vi "Configurator.vi"() -> ()   [LabVIEW 2017]
uses:
  Controls/Configurator Range Enum Type Def.ctl
  Controls/Configurator Rate Enum Type Def.ctl
  Controls/xlRange.ctl
panel:
  in  "Accelerometer Range":T1=enum."±8g"
  in  "First Erase?":bool
  in  "VISA":refnum<visa-resource-name>
  out "Error Out":errorcluster
  in  "Error In":errorcluster
  in  "ID":u8
  in  "Rate":T2=enum."52"
  in  "Angular Velocity Range":T3=enum."250 dps"
  # "Read and save measurement data before running this program!"
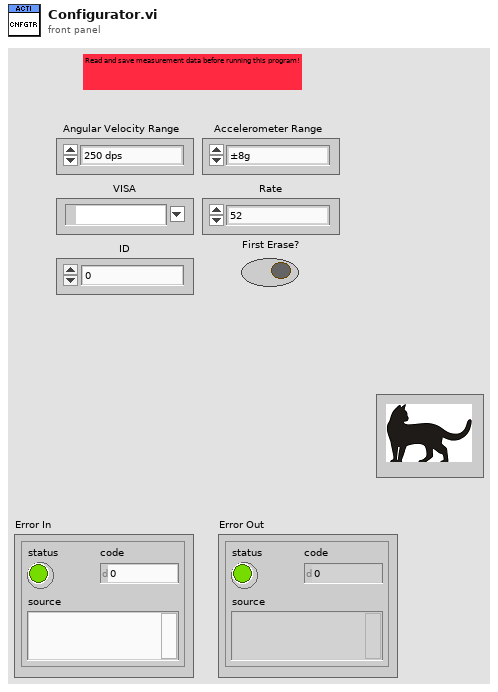
[diagram p1: front panel]
types:
  T1 = typedef "xlRange.ctl" = enum16{"±16g", "±8g", "±4g", "±2g"}
  T2 = typedef "Configurator Rate Enum Type Def.ctl" = enum16{"12,5", "208", "104", "52", "26", "Idle"}
  T3 = typedef "Configurator Range Enum Type Def.ctl" = enum16{"125 dps", "250 dps", "500 dps", "1000 dps", "2000 dps", ""}
  T4 = cluster{"Angular Velocity Range":T3, "Accelerometer Range":T1, "ID":u8, "VISA":refnum<visa-resource-name>, "First Erase?":bool, "xlRange":u8, "gyroRange":u8, "ODR":u8, "Time Bytes":string, "Rate":T2}
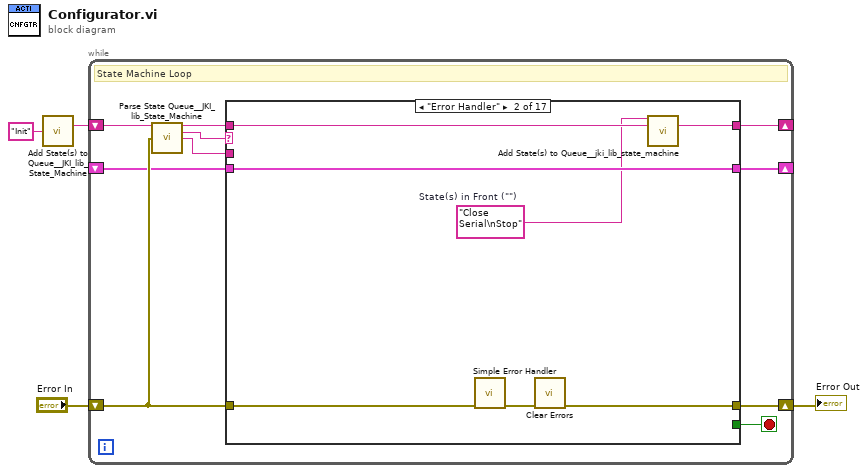
[diagram p0: block diagram]
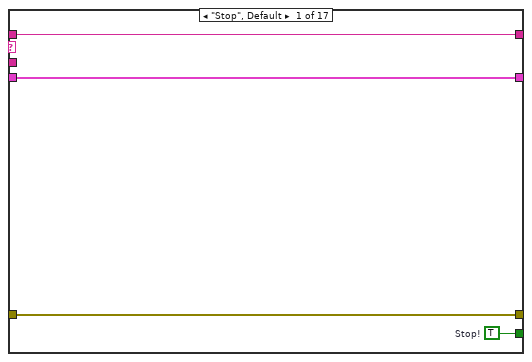
[diagram p2: hidden frame]
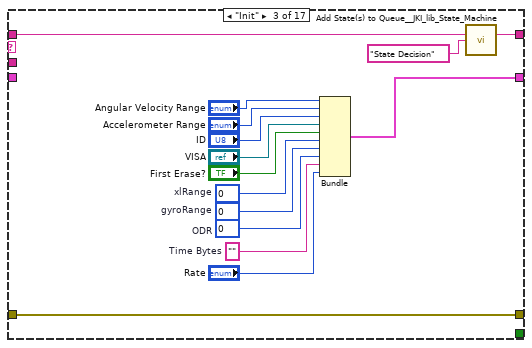
[diagram p3: hidden frame]
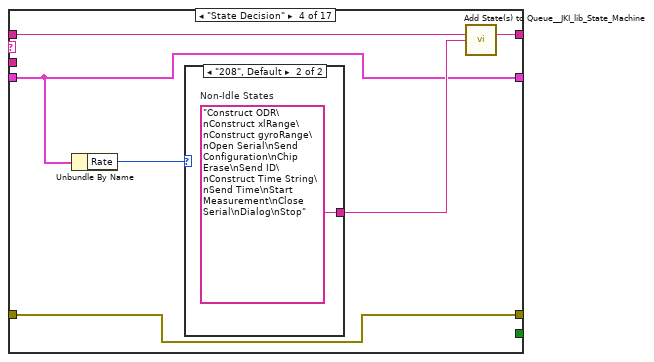
[diagram p4: hidden frame]
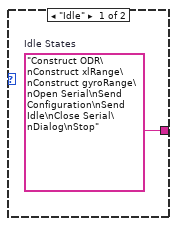
[diagram p5: hidden frame]
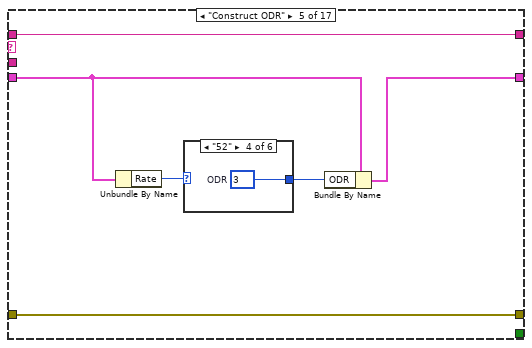
[diagram p6: hidden frame]
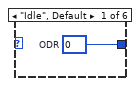
[diagram p7: hidden frame]
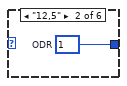
[diagram p8: hidden frame]
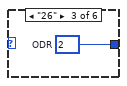
[diagram p9: hidden frame]
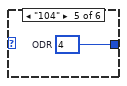
[diagram p10: hidden frame]
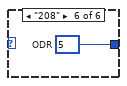
[diagram p11: hidden frame]
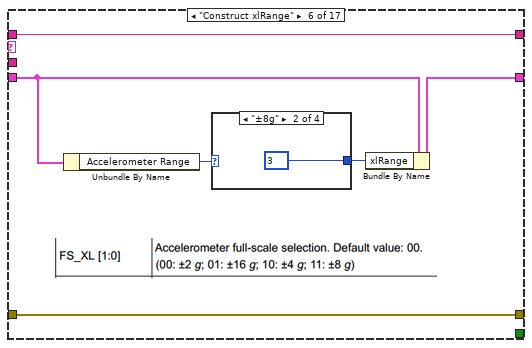
[diagram p12: hidden frame]
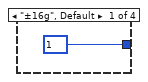
[diagram p13: hidden frame]
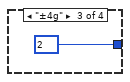
[diagram p14: hidden frame]
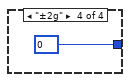
[diagram p15: hidden frame]
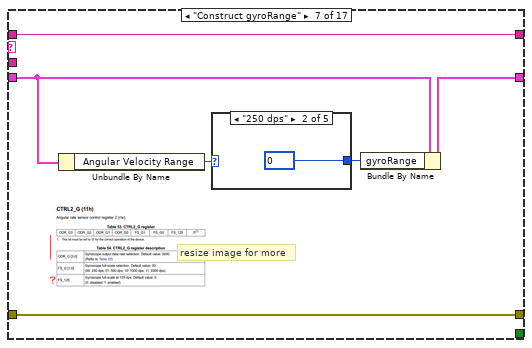
[diagram p16: hidden frame]
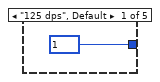
[diagram p17: hidden frame]
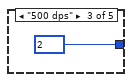
[diagram p18: hidden frame]
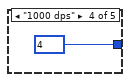
[diagram p19: hidden frame]
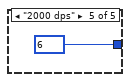
[diagram p20: hidden frame]
diagram:
  n1 = call <vilib>:"Add State(s) to Queue__JKI_lib_State_Machine.vi"("State(s) at Back (\"\")"="Init" ("State(s) at Back (\"\")")) -> ("States Out"=w2:string)  [unwired: 14 in]
  n2 = while {
    shift-right: [w13] -> w3
    shift-left: "Error In" -> [w14]
    shift-right: [w11] -> _
    shift-left: _ -> [w10]
    shift-right: [w6] -> _
    shift-left: w2 -> [w9]
    stop <- w12 stop-if-true
    # "State Machine Loop"
    n3 = call <vilib>:"Parse State Queue__JKI_lib_State_Machine.vi"("State Queue"=w9, "Error In (no error)"=w14) -> ("Remaining States"=w5:string, "Current State"=w8:string, "Arguments"=w7:string)  [unwired: 11 in]
    n4 = case shown="\"Error Handler\"" w8 {
      tunnel: w14 -> [w16 w25 w40 w42 w54 w66 w76 w87 w93 w114 w130 w140 w151 w157 w162 w175 w182]
      tunnel: [w16 w19 w40 w42 w54 w66 w76 w86 w100 w112 w122 w139 w150 w156 w161 w175 w182] -> w13
      tunnel: [w18 _ _ _ _ _ _ _ _ _ _ _ _ _ _ _ _] -> w12
      tunnel: [w17 w24 w31 w41 w50 w64 w74 w85 w101 w104 w129 w136 w149 w155 w160 w177 w180] -> w11
      tunnel: w10 -> [w17 w24 _ w41 w51 w65 w75 w85 w101 w104 w129 w143 w149 w155 w160 w177 w180]
      tunnel: w7 -> [_ _ _ _ _ _ _ _ _ _ _ _ _ _ _ _ _]
      tunnel: [w15 w23 w29 w46 w53 w63 w73 w83 w97 w102 w120 w132 w144 w152 w158 w174 w178] -> w6
      tunnel: w5 -> [w15 w22 w28 w45 w53 w63 w73 w83 w97 w102 w120 w132 w144 w152 w158 w174 w178]
      frame "Stop", Default {
        w18 = TRUE  # Stop!
      }
      frame "Error Handler" {
        w21 = "Close Serial\nStop"  # State(s) in Front ("")
        n5 = call <vilib>:"Simple Error Handler.vi"("error in (no error)"=w25) -> ("error out"=w20:errorcluster)  [unwired: 4 in, 4 out]
        n6 = call <vilib>:"Clear Errors.vi"("error in (no error)"=w20) -> ("error out"=w19:errorcluster)  [unwired: 5 in, 1 out]
        n7 = call <vilib>:"Add State(s) to Queue__jki_lib_state_machine.vi"("State(s) in Front (\"\")"=w21, "State(s) in (\"\")"=w22) -> ("States Out"=w23:string)  [unwired: 13 in]
      }
      frame "Init" {
        w30 = u8 0  # gyroRange
        w32 = ""  # Time Bytes
        w33 = u8 0  # ODR
        w34 = u8 0  # xlRange
        n8 = Bundle("Angular Velocity Range"="Angular Velocity Range", "Accelerometer Range"="Accelerometer Range", "ID"="ID", "VISA"="VISA", "First Erase?"="First Erase?", "xlRange"=w34, "gyroRange"=w30, "ODR"=w33, "Time Bytes"=w32, "Rate"="Rate") -> (w31:T4)  [unwired: 1 in]
        n9 = call <vilib>:"Add State(s) to Queue__JKI_lib_State_Machine.vi"("State(s) in (\"\")"=w28, "State(s) at Back (\"\")"="State Decision" ("State(s) at Back (\"\")")) -> ("States Out"=w29:string)  [unwired: 13 in]
      }
      frame "State Decision" {
        n10 = Unbundle By Name(w41) -> ("Rate"=w44:T2)
        n11 = case shown="\"208\", Default" w44 {
          tunnel: [w47 w48] -> w43
          frame "Idle" {
            w47 = "Construct ODR\nConstruct xlRange\nConstruct gyroRange\nOpen Serial\nSend Configuration\nSend Idle\nClose Serial\nDialog\nStop"  # Idle States
          }
          frame "208", Default {
            w48 = "Construct ODR\nConstruct xlRange\nConstruct gyroRange\nOpen Serial\nSend Configuration\nChip Erase\nSend ID\nConstruct Time String\nSend Time\nStart Measurement\nClose Serial\nDialog\nStop"  # Non-Idle States
          }
        }
        n12 = call <vilib>:"Add State(s) to Queue__JKI_lib_State_Machine.vi"("State(s) in (\"\")"=w45, "State(s) at Back (\"\")"=w43) -> ("States Out"=w46:string)  [unwired: 13 in]
      }
      frame "Construct ODR" {
        n13 = Unbundle By Name(w51) -> ("Rate"=w52:T2)
        n14 = case shown="\"52\"" w52 {
          tunnel: [w55 w56 w57 w58 w59 w60] -> w49
          frame "Idle", Default {
            w55 = u8 0  # ODR
          }
          frame "12,5" {
            w56 = u8 1  # ODR
          }
          frame "26" {
            w57 = u8 2  # ODR
          }
          frame "52" {
            w58 = u8 3  # ODR
          }
          frame "104" {
            w59 = u8 4  # ODR
          }
          frame "208" {
            w60 = u8 5  # ODR
          }
        }
        n15 = Bundle By Name(cluster=w51, "ODR"=w49) -> (w50:T4)
      }
      frame "Construct xlRange" {
        n16 = Unbundle By Name(w65) -> ("Accelerometer Range"=w62:T1)
        n17 = case shown="\"±8g\"" w62 {
          tunnel: [u8 1 u8 3 u8 2 u8 0] -> w61
          frame "±16g", Default {
          }
          frame "±8g" {
          }
          frame "±4g" {
          }
          frame "±2g" {
          }
        }
        n18 = Bundle By Name(cluster=w65, "xlRange"=w61) -> (w64:T4)
      }
      frame "Construct gyroRange" {
        # "resize image for more"
        n19 = Unbundle By Name(w75) -> ("Angular Velocity Range"=w72:T3)
        n20 = case shown="\"250 dps\"" w72 {
          tunnel: [u8 1 u8 0 u8 2 u8 4 u8 6] -> w71
          frame "125 dps", Default {
          }
          frame "250 dps" {
          }
          frame "500 dps" {
          }
          frame "1000 dps" {
          }
          frame "2000 dps" {
          }
        }
        n21 = Bundle By Name(cluster=w75, "gyroRange"=w71) -> (w74:T4)
      }
      frame "Open Serial" {
        w82 = u32 6000000  # Baud rate
        n22 = Unbundle By Name(w85) -> ("VISA"=w84:refnum<visa-resource-name>)
        n23 = call "Init_VSP.vi"("error in"=w87, "Baud rate"=w82, "VISA resource name"=w84) -> ("error out"=w86:errorcluster)  [unwired: 7 in, 1 out]
      }
      frame "Send Configuration" {
        w90 = FALSE  # Prepend Size?
        w88 = "*C"  # Configure Command
        n24 = Unbundle By Name(w101) -> ("VISA"=w99:refnum<visa-resource-name>, "ODR"=w94:u8, "xlRange"=w96:u8, "gyroRange"=w95:u8)
        n25 = Build Array(w94, w96, w95) -> (w91:u8[])
        n26 = Flatten To String(anything=w91, prepend array or string size? (T)=w90, error in (no error)=w93) -> (data string=w89:string, error out=w92:errorcluster)  [unwired: 1 in, 1 out]
        n27 = Concatenate Strings(w88, w89) -> (w98:string)
        n28 = call "Write Serial One by One With Echo.vi"("String"=w98, "Error In"=w92, "VISA In"=w99) -> ("Error Out"=w100:errorcluster)  [unwired: 7 in, 1 out]
      }
      frame "Chip Erase" {
        w108 = "*1*Y"  # First Erase
        w107 = "*Y"  # Chip Erase Command
        n29 = Unbundle By Name(w104) -> ("First Erase?"=w103:bool)
        n30 = Unbundle By Name(w104) -> ("VISA"=w106:refnum<visa-resource-name>)
        n31 = Select(t=w108, s=w103, f=w107) -> (s? t:f=w105:string)
        n32 = call "Write Serial One by One With Echo.vi"("String"=w105, "Error In"=w114, "VISA In"=w106) -> ("Error Out"=w113:errorcluster, "VISA Out"=w110:refnum<visa-resource-name>)  [unwired: 7 in]
        n33 = for {
          N: 4 -> [_]
          shift-right: [w118] -> w112
          shift-left: w113 -> [w119]
          tunnel: u32 1 ("Requested byte cout") -> [w117]
          tunnel: w110 -> [w116]
          tunnel: [w115] -> _ mode=indexing
          n34 = call "Read_VSP.vi"("error in"=w119, "Requested byte count"=w117, "VISA resource name"=w116) -> ("error out"=w118:errorcluster, "String"=w115:string)  [unwired: 1 in, 2 out]
        }
      }
      frame "Send ID" {
        w126 = FALSE  # Prepend Size?
        w131 = "*D"  # Send ID Command
        n35 = Unbundle By Name(w129) -> ("ID"=w121:u8, "VISA"=w128:refnum<visa-resource-name>)
        n36 = call "Write Serial One by One With Echo.vi"("String"=w131, "Error In"=w130, "VISA In"=w128) -> ("Error Out"=w127:errorcluster, "VISA Out"=w124:refnum<visa-resource-name>)  [unwired: 7 in]
        n37 = Flatten To String(anything=w121, prepend array or string size? (T)=w126, error in (no error)=w127) -> (data string=w123:string, error out=w125:errorcluster)  [unwired: 1 in, 1 out]
        n38 = call "Write_VSP.vi"("error in"=w125, "String"=w123, "VISA resource name"=w124) -> ("error out"=w122:errorcluster)  [unwired: 2 in, 2 out]
      }
      frame "Construct Time String" {
        w133 = 4 ("offset (0)")
        w137 = FALSE  # Prepend Size?
        n39 = Get Date/Time In Seconds() -> (seconds since 1Jan1904=w142:timestamp)
        n40 = To Double Precision Float(number=w142) -> (double precision float=w141:dbl)
        n41 = To Unsigned Quad Integer(1:w141) -> (0:w138:u64)
        n42 = Flatten To String(anything=w138, prepend array or string size? (T)=w137, error in (no error)=w140) -> (data string=w134:string, error out=w139:errorcluster)  [unwired: 1 in, 1 out]
        n43 = String Subset(string=w134, offset (0)=w133, length (rest)=w133) -> (substring=w135:string)
        n44 = Bundle By Name(cluster=w143, "Time Bytes"=w135) -> (w136:T4)
      }
      frame "Send Time" {
        w148 = "*T"  # Set Time Command
        n45 = Unbundle By Name(w149) -> ("Time Bytes"=w147:string, "VISA"=w146:refnum<visa-resource-name>)
        n46 = Concatenate Strings(w148, w147) -> (w145:string)
        n47 = call "Write Serial One by One With Echo.vi"("String"=w145, "Error In"=w151, "VISA In"=w146) -> ("Error Out"=w150:errorcluster)  [unwired: 7 in, 1 out]
      }
      frame "Start Measurement" {
        w153 = "*S"  # Start Command
        n48 = Unbundle By Name(w155) -> ("VISA"=w154:refnum<visa-resource-name>)
        n49 = call "Write Serial One by One With Echo.vi"("String"=w153, "Error In"=w157, "VISA In"=w154) -> ("Error Out"=w156:errorcluster)  [unwired: 7 in, 1 out]
      }
      frame "Send Idle" {
        w164 = u8 27  # Esc Character
        w165 = u32 1  # Requested byte cout
        n50 = Unbundle By Name(w160) -> ("VISA"=w159:refnum<visa-resource-name>)
        n51 = call "Write_VSP.vi"("error in"=w162, "String"="*", "VISA resource name"=w159) -> ("error out"=w171:errorcluster, "duplicate VISA resource name"=w170:refnum<visa-resource-name>)  [unwired: 2 in, 1 out]
        n52 = Flatten To String(anything=w164) -> (data string=w163:string)  [unwired: 3 in, 2 out]
        n53 = call "Read_VSP.vi"("error in"=w171, "Requested byte count"=w165, "VISA resource name"=w170) -> ("error out"=w167:errorcluster, "duplicate VISA resource name"=w166:refnum<visa-resource-name>)  [unwired: 1 in, 2 out]
        n54 = call "Write_VSP.vi"("error in"=w167, "String"=w163, "VISA resource name"=w166) -> ("error out"=w168:errorcluster, "duplicate VISA resource name"=w169:refnum<visa-resource-name>)  [unwired: 2 in, 1 out]
        n55 = call "Read_VSP.vi"("error in"=w168, "Requested byte count"=w165, "VISA resource name"=w169) -> ("error out"=w161:errorcluster)  [unwired: 1 in, 3 out]
      }
      frame "Close Serial" {
        n56 = Unbundle By Name(w177) -> ("VISA"=w176:refnum<visa-resource-name>)
        n57 = call "Close_VSP.vi"("VISA resource name"=w176) -> ("error out"=w173:errorcluster)  [unwired: 6 in]
        n58 = call <vilib>:"Clear Errors.vi"("error in (no error)"=w173) -> ()  [unwired: 5 in, 2 out]
      }
      frame "Dialog" {
        n59 = Unbundle By Name(w180) -> ("Rate"=w181:T2)
        n60 = case shown="\"12,5\", Default" w181 {
          tunnel: ["Idle command sent.\nRemove device now." ("message") "Start command sent.\nRemove device now." ("message")] -> w179
          frame "Idle" {
          }
          frame "12,5", Default {
          }
        }
        n61 = One Button Dialog(message=w179) -> ()  [unwired: 1 in, 1 out]
      }
    }
  }
  "Error Out" <- w3
